vi "Initialize Interaction Map (incoming).vi"(8 "error in":errorcluster, 9 "interaction name":string, 10 "incoming interactions":map{string, map{string, i32}}(c390), 11 "in_interaction map in":T1) -> (0 "error out":errorcluster, 3 "in_interaction map out":T1)   [LabVIEW 2019, in "HLA Custom Device Engine.lvlib"]
uses:
  HLA Custom Device Engine.lvlib
  _typedefs/map_interaction_value.ctl
  _typedefs/map_attr_param_data.ctl
  <vilib>/addons/hla/helpers/phvm.lvlib
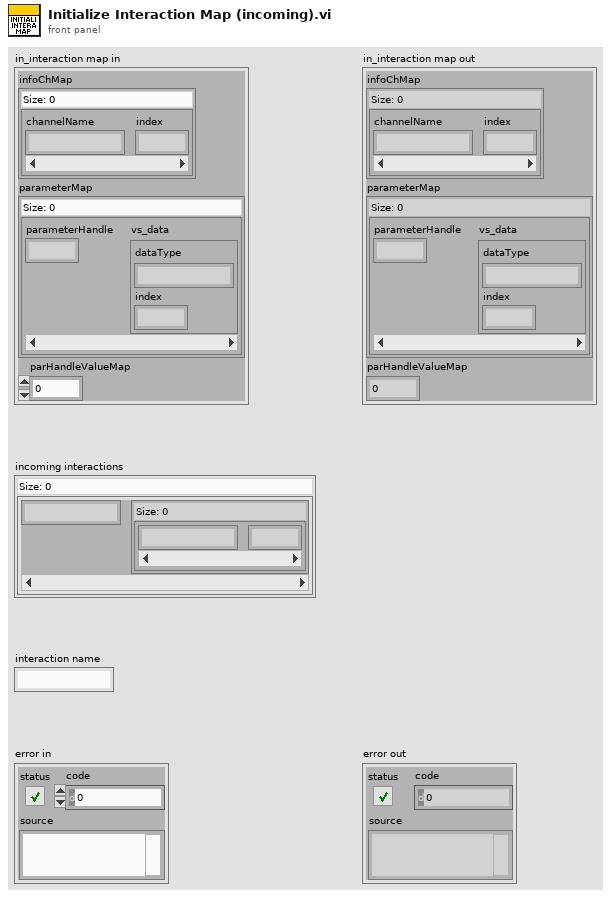
[diagram p1: front panel]
types:
  T1 = typedef "HLA Custom Device Engine.lvlib/map_interaction_value.ctl" = cluster{"infoChMap":map{string, i32}, "parameterMap":map{u64, T2}, "parHandleValueMap":u64}
  T2 = typedef "HLA Custom Device Engine.lvlib/map_attr_param_data.ctl" = cluster{"dataType":string, "index":i32}
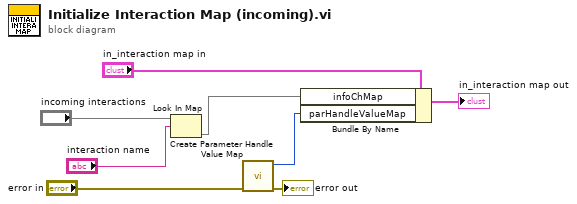
[diagram p0: block diagram]
diagram:
  n1 = Look In Map(map="incoming interactions", key="interaction name") -> (value=w6:map{string, i32})  [unwired: 1 in, 1 out]
  n2 = call <vilib>:"Create Parameter Handle Value Map.vi"("error in"="error in") -> ("error out"=→"error out":errorcluster, "parHandleValueMap"=w1:u64)  [unwired: 9 in]
  n3 = Bundle By Name(cluster="in_interaction map in", "infoChMap"=w6, "parHandleValueMap"=w1) -> (→"in_interaction map out":T1)
